vi "Convert High Voltage and Return Channel to Raw String.vi"(9 "Return Channels":i32[](array[numeric]), 10 "High Voltage Channels":i32[](array[numeric])) -> (2 "Command Raw String":string)   [LabVIEW 2014, in "Associated Research SC6540.lvlib"]
doc: "Convert channel array of high voltage and generate the raw string."
uses:
  <instrlib>/Associated Research SC6540/Associated Research SC6540.lvlib
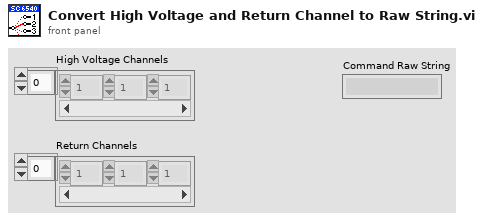
[diagram p1: front panel]
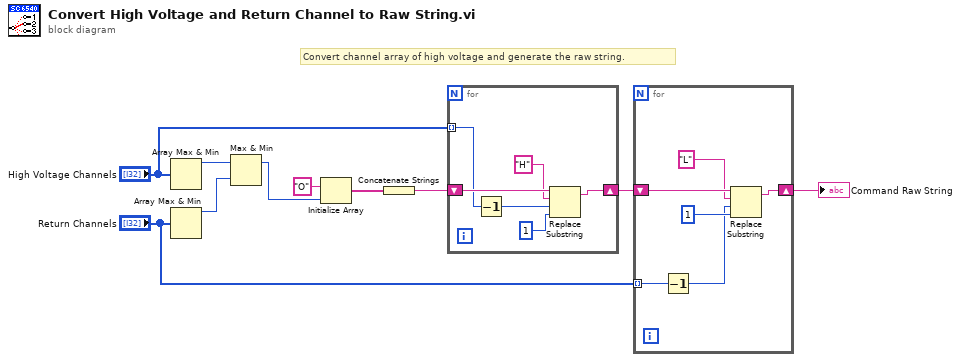
[diagram p0: block diagram]
diagram:
  # "Convert channel array of high voltage and generate the raw string."
  n1 = Array Max & Min(array="High Voltage Channels") -> (max value=w10:i32)  [unwired: 3 out]
  n2 = Array Max & Min(array="Return Channels") -> (max value=w9:i32)  [unwired: 3 out]
  n3 = Max & Min(x=w10, y=w9) -> (max(x,y)=w3:i32)  [unwired: 1 out]
  n4 = Initialize Array("O" ("element"), w3) -> (w4:string[])
  n5 = Concatenate Strings(w4) -> (w1:string)
  n6 = for {
    shift-right: [w16] -> w6
    shift-left: w1 -> [w15]
    tunnel: "High Voltage Channels" -> [w12] mode=indexing
    n7 = Decrement(x=w12) -> (x-1=w11:i32)
    n8 = Replace Substring(2:1 ("length (len. of substring)"), 3:w11, 4:"H" ("new element/subarray"), 5:w15) -> (1:w16:string)  [unwired: 1 out]
  }
  n9 = for {
    shift-right: [w22] -> w5
    shift-left: w6 -> [w21]
    tunnel: "Return Channels" -> [w18] mode=indexing
    n10 = Decrement(x=w18) -> (x-1=w17:i32)
    n11 = Replace Substring(2:1 ("length (len. of substring)"), 3:w17, 4:"L" ("new element/subarray"), 5:w21) -> (1:w22:string)  [unwired: 1 out]
  }
  "Command Raw String" <- w5
